vi "step2 SolveLowerRightCornerPiece.vi"(8 "error in (no error)":errorcluster, 10 "operation queue":refnum<queue>, 11 "cube in":T1) -> (0 "error out":errorcluster, 2 "operation queue out":refnum<queue>, 3 "cube out":T1)   [LabVIEW 2011]
doc: "Rotate cube as necessary so that the top middle piece matches the desired start colour.\n\nNo transformations are done in this VI, the operations are loaded on the the operation queue bus."
uses:
  Typedef/cube.ctl
  Typedef/face.ctl
  Typedef/main state.ctl
  Typedef/operation.ctl
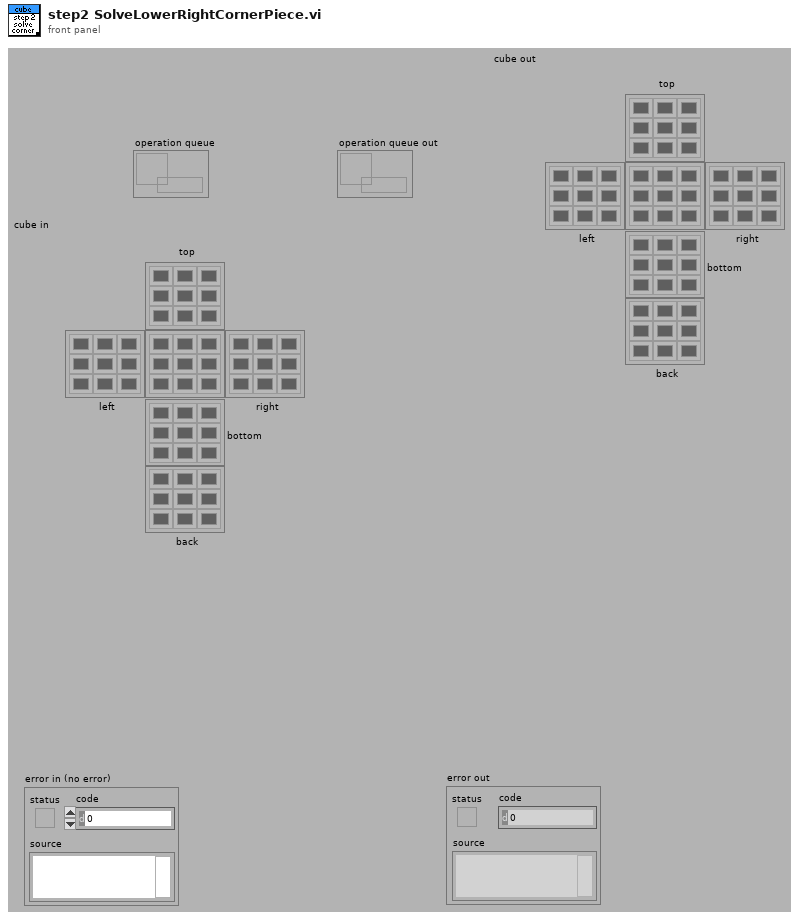
[diagram p1: front panel]
types:
  T1 = typedef "cube.ctl" = cluster{"top":T2, "left":T2, "right":T2, "bottom":T2, "back":T2, "front":T2}
  T2 = typedef "face.ctl" = u32[][]
  T3 = typedef "operation.ctl" = enum16{"nop", "T+", "T-", "F+", "F-", "L+", "L-", "R+", "R-", "B+", "B-", "<--", "-->", "^", "V"}
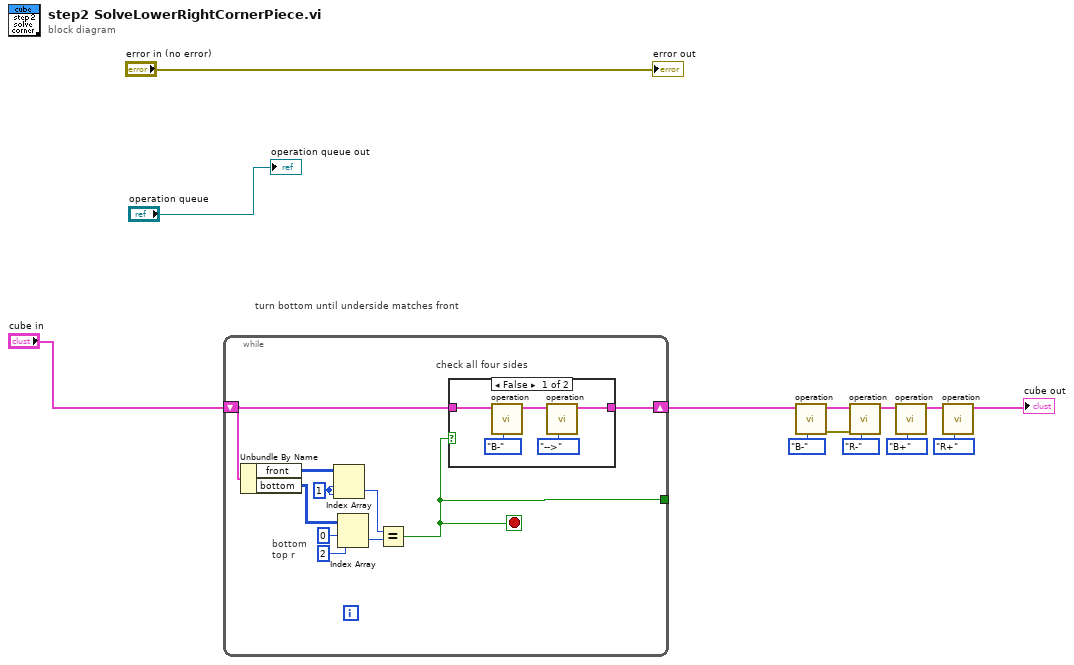
[diagram p0: block diagram]
diagram:
  # "turn bottom until underside matches front"
  n1 = while {
    shift-right: [w22] -> w4
    shift-left: "cube in" -> [w23]
    tunnel: [w17] -> _
    stop <- w17 stop-if-true
    w16 = 1 ("index (row)")
    # "bottom\ntop r"
    # "check all four sides"
    n2 = Unbundle By Name(w23) -> ("front"=w15:T2, "bottom"=w18:T2)
    n3 = Index Array(array=w15, index (row)=w16, index (col)=w16) -> (element=w14:u32)
    n4 = Index Array(array=w18, index (row)=0, index (col)=2 ("index (row)")) -> (element=w19:u32)
    n5 = Equal?(x=w14, y=w19) -> (x = y?=w17:bool)
    n6 = case shown="False" w17 {
      tunnel: w23 -> [w26 w29]
      tunnel: [w24 w29] -> w22
      frame False {
        n7 = call "operation.vi"("operation"=operation."B-", "cube in"=w26) -> ("cube out"=w25:T1)  [unwired: 8 in, 1 out]
        n8 = call "operation.vi"("operation"=operation."-->", "cube in"=w25) -> ("cube out"=w24:T1)  [unwired: 8 in, 1 out]
      }
      frame True {
      }
    }
  }
  n9 = call "operation.vi"("operation"=operation."B-", "cube in"=w4) -> ("error out"=w8:errorcluster, "cube out"=w7:T1)  [unwired: 8 in]
  n10 = call "operation.vi"("operation"=operation."R-", "error in (no error)"=w8, "cube in"=w7) -> ("cube out"=w3:T1)  [unwired: 7 in, 1 out]
  n11 = call "operation.vi"("operation"=operation."B+", "cube in"=w3) -> ("cube out"=w2:T1)  [unwired: 8 in, 1 out]
  n12 = call "operation.vi"("operation"=operation."R+", "cube in"=w2) -> ("cube out"=→"cube out":T1)  [unwired: 8 in, 1 out]
  "error out" <- "error in (no error)"
  "operation queue out" <- "operation queue"
